vi "Home_Single_Device_COMPort_Free_Text_Commands.vi"   [LabVIEW 2017]
uses:
  U:/UDocuments/Thorlabs.Elliptec.ELLO_DLL.dll
  Thorlabs.Elliptec.ELLO_DLL.dll
panel:
  # "Notes:"
  # "This VI does not require you to use specific hardware. Any elliptec device is compatible and can they can be running \"Daisy-Chained\" \nor through the ELLB Control Bus Distributor. The maximum number of devices it can search through on a single COM port is 16.\nThe stages can not share the same address as this will cause confusion and only one device will be displayed, with a serial number \nwhich corresponds to neither stage.\n\nIf, when running the VI for the first time, you get a popup as illustrated below, then click Browse and navigate to the \nThorlabs.Elliptec.ELLO_DLL.dll file in the ELLO software installation directory. This can be copied to the folder you are \nrunning the VI from."
  # "Thorlabs Hardware: ELL6, ELL9, ELL14, ELL17, ELL18, ELLB \nhttps://www.thorlabs.com/thorproduct.cfm?partnumber=ELL17\n\nDescription: This VI will enable you to control an Elliptec stage by sending free text commands directly to a stage on at a specific COM port.\nYou will need to know the COM port your device is using and the address of the stage. \n\nBy default this address will be 0 unless changed by a user. It can be any value in Hex from 0 to F. If the device address is unknown then this is most easily found through the ELLO software:\n \nhttps://www.thorlabs.com/software_pages/ViewSoftwarePage.cfm?Code=ELL"
  # "Instructions:"
  # "1) Connect your device to the USB Interface board via the ribbon cable. \n2) Connect power to the board and wait for approximately 10 seconds. As soon as the stage has power it will attempt a frequency search.\n     If the power is insufficient the board will not find the correct operating frequencies. This is why the USB is attached last.\n3) Connect the interface board to the PC via the USB cable.\n4) Open the VI, then enter the address of the device being used and select the homing direction you wish to use.\n5) Run the VI"
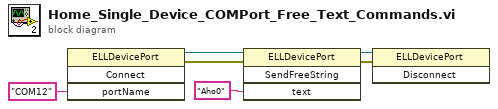
[diagram p0: block diagram]
diagram:
  n1 = invoke class="ELLDevicePort" method="Connect"("portName"="COM12") -> (reference out=w4:refnum<k24>, error out=w2:errorcluster)  [unwired: 3 in, 2 out]
  n2 = invoke class="ELLDevicePort" method="SendFreeString"(reference=w4, error in=w2, "text"="Aho0") -> (reference out=w1:refnum<k24>, error out=w3:errorcluster)  [unwired: 1 in, 2 out]
  n3 = invoke class="ELLDevicePort" method="Disconnect"(reference=w1, error in=w3) -> ()  [unwired: 1 in, 3 out]
